vi "Get Response Fit.vi"(8 "error in (no error)":errorcluster, 11 "Sinusoidal Fit in":refnum<class "Sinusoidal Fit.lvclass">) -> (0 "error out":errorcluster, 2 "Fit out":dbl[](array[numeric]), 3 "Sinusoidal Fit out":refnum<class "Sinusoidal Fit.lvclass">)   [LabVIEW 2013, in "Sinusoidal Fit.lvclass"]
uses:
  Sinusoidal Fit.lvclass
  Sinusoidal Fit.lvclass/Sinusoidal Fit.ctl
  <vilib>/measure/NI_MABase.lvlib
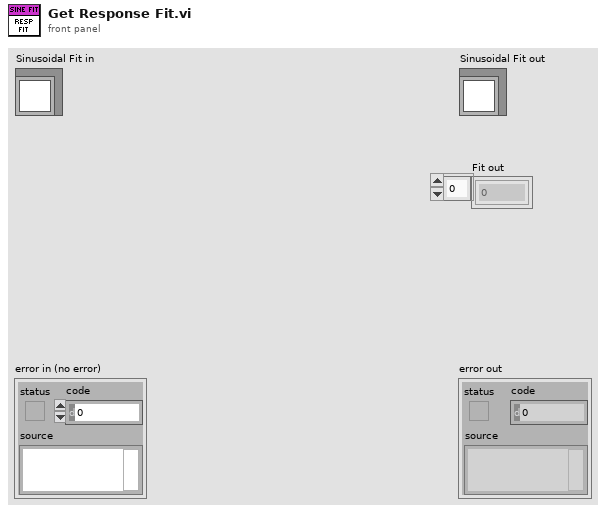
[diagram p1: front panel]
types:
  T1 = typedef "Typedef - Sinusoidal Fit Coefficients.ctl" = cluster{"Offset":dbl, "Gain":dbl, "Phase":dbl, "Freq":dbl}
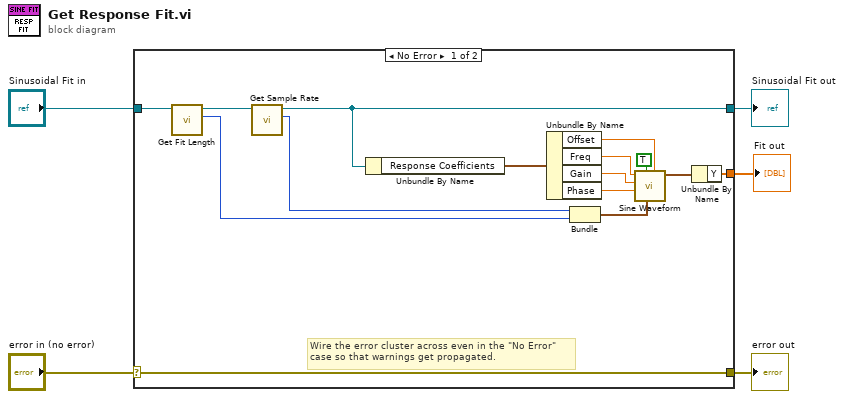
[diagram p0: block diagram]
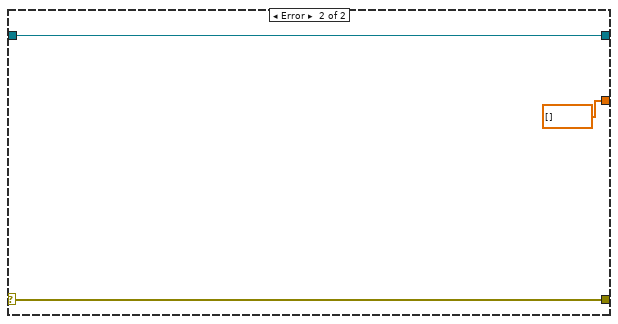
[diagram p2: hidden frame]
diagram:
  n1 = case shown="No Error" "error in (no error)" {
    selector: "error in (no error)" -> [w20 w23]
    tunnel: [w20 w23] -> w4
    tunnel: [w8 w22] -> w2
    tunnel: "Sinusoidal Fit in" -> [w10 w22]
    tunnel: [w11 dbl[] [] ("Y")] -> w1
    frame No Error {
      # "Wire the error cluster across even in the \"No Error\"\ncase so that warnings get propagated."
      n2 = call-dynamic "Get Fit Length.vi"("Abstract Fit in"=w10) -> ("Length"=w7:i32, "Abstract Fit out"=w9:refnum<class "Sinusoidal Fit.lvclass">)  [unwired: 8 in, 1 out]
      n3 = call-dynamic "Get Sample Rate.vi"("Abstract Fit in"=w9) -> ("Sample Rate"=w6:i32, "Abstract Fit out"=w8:refnum<class "Sinusoidal Fit.lvclass">)  [unwired: 8 in, 1 out]
      n4 = Unbundle By Name(w8) -> ("Response Coefficients"=w19:T1)
      n5 = Unbundle By Name(w19) -> ("Offset"=w18:dbl, "Freq"=w16:dbl, "Gain"=w15:dbl, "Phase"=w14:dbl)
      n6 = Bundle("Sample Rate"=w6, "Length"=w7) -> (w12:cluster{"Sample Rate":i32, "Length":i32})  [unwired: 1 in]
      n7 = call <vilib>:"Sine Waveform.vi"("offset"=w18, "sampling info"=w12, "reset signal"=TRUE, "phase"=w14, "amplitude"=w15, "frequency"=w16) -> ("signal out"=w13:waveform(dbl))  [unwired: 4 in, 1 out]
      n8 = Unbundle By Name(w13) -> ("Y"=w11:dbl[])
    }
    frame Error {
    }
  }
  "error out" <- w4
  "Sinusoidal Fit out" <- w2
  "Fit out" <- w1
